vi "循环数据分析.vi"(8 "ÃðãÐÖµ":i32=200, 9 "ÁÁãÐÖµ":i32=400, 10 "颜色选择":enum16{"红", "绿", "蓝", "白", "黄", "çúçêÉ«"}(ring), 11 "循环数据":u16[][](array[numeric])) -> (0 "i":u16, 1 "B":u16, 2 "G":u16, 3 "R":u16, 4 "闪烁？":bool, 5 "颜色结果":bool)   [LabVIEW 2015]
panel:
  out "灭":i32=6
  out "亮":i32=9
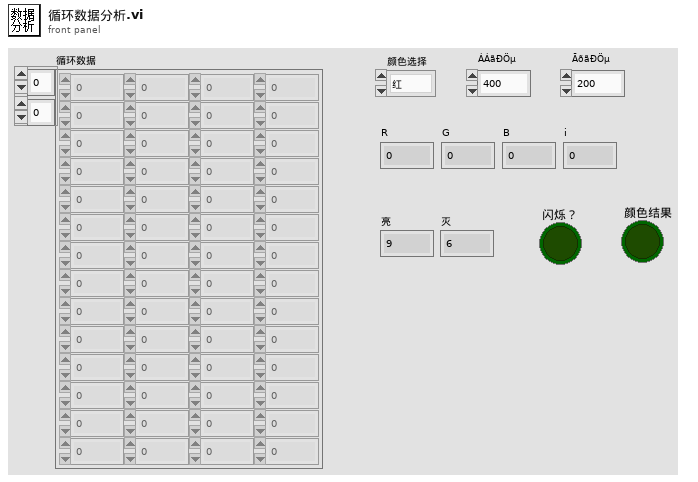
[diagram p1: front panel]
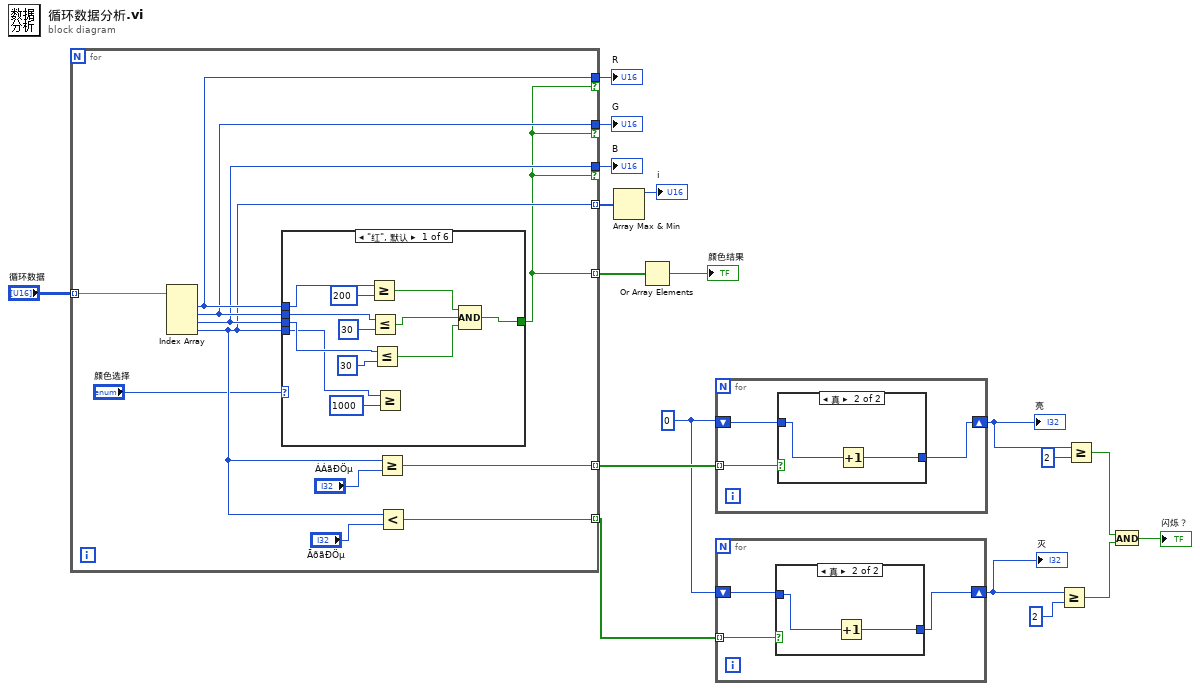
[diagram p0: block diagram]
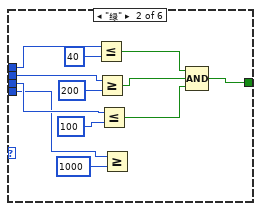
[diagram p4: hidden frame]
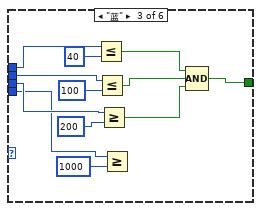
[diagram p5: hidden frame]
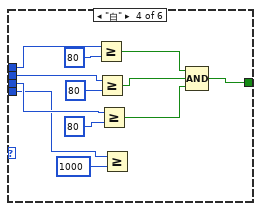
[diagram p6: hidden frame]
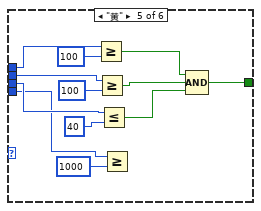
[diagram p7: hidden frame]
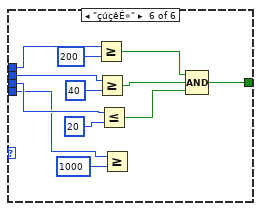
[diagram p8: hidden frame]
diagram:
  w10 = 0
  n1 = for {
    tunnel: "循环数据" -> [w29] mode=indexing
    tunnel: [w28] -> w3 if=w20
    tunnel: [w27] -> w2 if=w20
    tunnel: [w26] -> w1 if=w20
    tunnel: [w23] -> w9 mode=indexing
    tunnel: [w22] -> w11 mode=indexing
    tunnel: [w21] -> w7 mode=indexing
    tunnel: [w20] -> w4 mode=indexing
    n2 = Index Array(array=w29) -> (element #1=w28:u16, element #2=w27:u16, element #3=w26:u16, element #4=w21:u16)  [unwired: 4 in]
    n3 = case shown="\"红\", 默认" "颜色选择" {
      tunnel: w28 -> [w41 w53 w65 w77 w89 w101]
      tunnel: w27 -> [w39 w51 w63 w75 w87 w99]
      tunnel: w26 -> [w37 w49 w61 w73 w85 w97]
      tunnel: w21 -> [w31 w43 w55 w67 w79 w91]
      tunnel: [w32 w44 w56 w68 w80 w92] -> w20
      frame "红", Default {
        n4 = Greater Or Equal?(x=w41, y=u32 200) -> (x >= y?=w35:bool)
        n5 = Less Or Equal?(x=w39, y=u32 30) -> (x <= y?=w34:bool)
        n6 = Less Or Equal?(x=w37, y=u32 30) -> (x <= y?=w33:bool)
        n7 = Greater Or Equal?(x=w31, y=u32 1000) -> ()  [unwired: 1 out]
        n8 = Compound Arithmetic op=AND ("复合运算")(w35, w34, w33) -> (w32:bool)
      }
      frame "绿" {
        n9 = Less Or Equal?(x=w53, y=u32 40) -> (x <= y?=w47:bool)
        n10 = Greater Or Equal?(x=w51, y=u32 200) -> (x >= y?=w46:bool)
        n11 = Less Or Equal?(x=w49, y=u32 100) -> (x <= y?=w45:bool)
        n12 = Greater Or Equal?(x=w43, y=u32 1000) -> ()  [unwired: 1 out]
        n13 = Compound Arithmetic op=AND ("复合运算")(w47, w46, w45) -> (w44:bool)
      }
      frame "蓝" {
        n14 = Less Or Equal?(x=w65, y=u32 40) -> (x <= y?=w59:bool)
        n15 = Less Or Equal?(x=w63, y=u32 100) -> (x <= y?=w58:bool)
        n16 = Greater Or Equal?(x=w61, y=u32 200) -> (x >= y?=w57:bool)
        n17 = Greater Or Equal?(x=w55, y=u32 1000) -> ()  [unwired: 1 out]
        n18 = Compound Arithmetic op=AND ("复合运算")(w59, w58, w57) -> (w56:bool)
      }
      frame "白" {
        n19 = Greater Or Equal?(x=w77, y=u32 80) -> (x >= y?=w71:bool)
        n20 = Greater Or Equal?(x=w75, y=u32 80) -> (x >= y?=w70:bool)
        n21 = Greater Or Equal?(x=w73, y=u32 80) -> (x >= y?=w69:bool)
        n22 = Greater Or Equal?(x=w67, y=u32 1000) -> ()  [unwired: 1 out]
        n23 = Compound Arithmetic op=AND ("复合运算")(w71, w70, w69) -> (w68:bool)
      }
      frame "黄" {
        n24 = Greater Or Equal?(x=w89, y=u32 100) -> (x >= y?=w83:bool)
        n25 = Greater Or Equal?(x=w87, y=u32 100) -> (x >= y?=w82:bool)
        n26 = Less Or Equal?(x=w85, y=u32 40) -> (x <= y?=w81:bool)
        n27 = Greater Or Equal?(x=w79, y=u32 1000) -> ()  [unwired: 1 out]
        n28 = Compound Arithmetic op=AND ("复合运算")(w83, w82, w81) -> (w80:bool)
      }
      frame "çúçêÉ«" {
        n29 = Greater Or Equal?(x=w101, y=u32 200) -> (x >= y?=w95:bool)
        n30 = Greater Or Equal?(x=w99, y=u32 40) -> (x >= y?=w94:bool)
        n31 = Less Or Equal?(x=w97, y=u32 20) -> (x <= y?=w93:bool)
        n32 = Greater Or Equal?(x=w91, y=u32 1000) -> ()  [unwired: 1 out]
        n33 = Compound Arithmetic op=AND ("复合运算")(w95, w94, w93) -> (w92:bool)
      }
    }
    n34 = Greater Or Equal?(x=w21, y="ÁÁãÐÖµ") -> (x >= y?=w22:bool)
    n35 = Less?(x=w21, y="ÃðãÐÖµ") -> (x < y?=w23:bool)
  }
  "R" <- w3
  "G" <- w2
  "B" <- w1
  n36 = Array Max & Min(array=w7) -> (max value=→"i":u16)  [unwired: 3 out]
  n37 = Or Array Elements(Boolean array=w4) -> (logical OR=→"颜色结果":bool)
  n38 = for {
    tunnel: w11 -> [w104] mode=indexing
    shift-right: [w102] -> w16
    shift-left: w10 -> [w103]
    n39 = case shown="真" w104 {
      tunnel: w103 -> [w105 w107]
      tunnel: [w105 w106] -> w102
      frame False {
      }
      frame True {
        n40 = Increment(x=w107) -> (x+1=w106:i32)
      }
    }
  }
  "亮" <- w16
  n41 = for {
    shift-right: [w108] -> w8
    shift-left: w10 -> [w110]
    tunnel: w9 -> [w109] mode=indexing
    n42 = case shown="真" w109 {
      tunnel: w110 -> [w111 w113]
      tunnel: [w111 w112] -> w108
      frame False {
      }
      frame True {
        n43 = Increment(x=w113) -> (x+1=w112:i32)
      }
    }
  }
  "灭" <- w8
  n44 = Greater Or Equal?(x=w8, y=2) -> (x >= y?=w13:bool)
  n45 = Greater Or Equal?(x=w16, y=2) -> (x >= y?=w12:bool)
  n46 = And(x=w12, y=w13) -> (x .and. y?=→"闪烁？":bool)
